vi "GenC37.118Cmd.vi"(7 "Function":T1=enum."Send CFG-2 file", 8 "error in (no error)":errorcluster, 11 "PMUClass":refnum<class "C37.118 PMU.lvclass">) -> (0 "error out":errorcluster, 2 "Command":string, 3 "PMUClass":refnum<class "C37.118 PMU.lvclass">)   [LabVIEW 2018, in "SensorPlugins.lvlib" / "C37.118 PMU.lvclass"]
uses:
  C37.118 PMU.lvclass
  Typedef/eCmdTypes.ctl
  C37.118 PMU.lvclass/C37.118 PMU.ctl
  Accessors/Read PMUComms.vi
panel:
  out "output array":u8[](array[numeric])=[68, 65, 13, 10, 0, 1, 67, 168, 27, 80, 0, 1, 0, 0, 0, 1, 94, 87] format="%x"
  out "*(type *) &x":u8[](array[numeric]) format="%x"
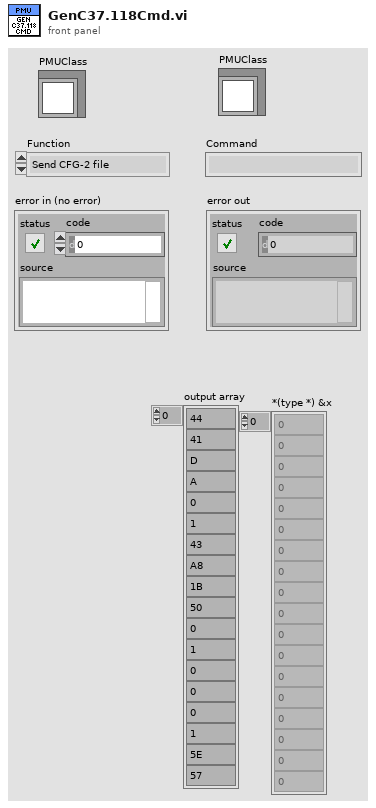
[diagram p1: front panel]
types:
  T1 = typedef "SensorPlugins.lvlib/C37.118 PMU.lvclass/eCmdTypes.ctl" = enum16{"Stop realtime data", "Start realtime data", "Send HDR file", "Send CFG-1 file", "Send CFG-2 file"}
  T2 = typedef "SensorPlugins.lvlib/C37.118 PMU.lvclass/PMUComms.ctl" = cluster{"PMU IP Address":string, "CMD Comms Type":T3, "Data Comms Type":T3, "CMD Port":u16, "Data Port":u16, "PMU ID":u16}
  T3 = typedef "SensorPlugins.lvlib/C37.118 PMU.lvclass/eCommsType.ctl" = enum16{"TCP", "UDP", "USB", "GPIB"}
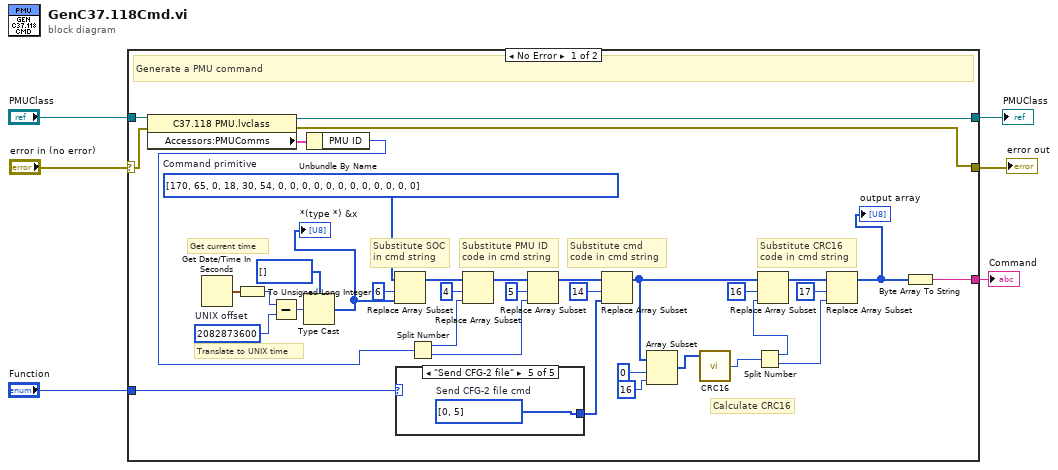
[diagram p0: block diagram]
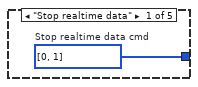
[diagram p2: hidden frame]
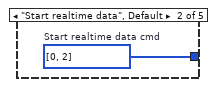
[diagram p3: hidden frame]
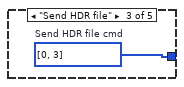
[diagram p4: hidden frame]
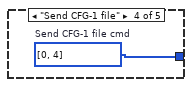
[diagram p5: hidden frame]
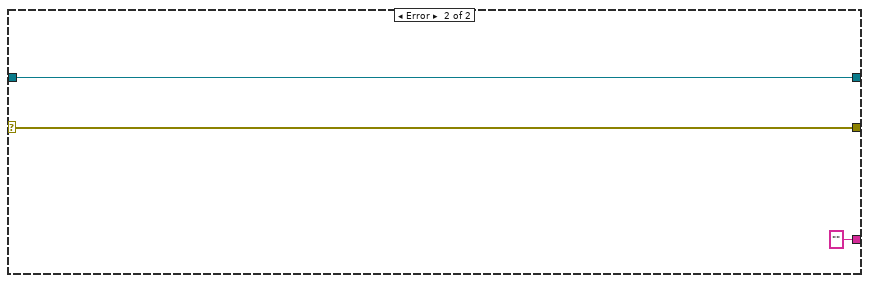
[diagram p6: hidden frame]
diagram:
  n1 = case shown="No Error" "error in (no error)" {
    selector: "error in (no error)" -> [w11 w50]
    tunnel: [w9 w50] -> w5
    tunnel: "PMUClass" -> [w14 w49]
    tunnel: [w10 w49] -> w3
    tunnel: "Function" -> [w8 _]
    tunnel: [w7 "" ("string")] -> w1
    frame No Error {
      w25 = u32 2082873600  # UNIX offset
      w22 = u8[] [170, 65, 0, 18, 30, 54, 0, 0, 0, 0, 0, 0, 0, 0, 0, 0, 0, 0]  # Command primitive
      # "Translate to UNIX time"
      # "Substitute SOC in cmd string"
      # "Get current time"
      # "Calculate CRC16"
      # "Substitute CRC16 code in cmd string"
      # "Substitute cmd code in cmd string"
      # "Substitute PMU ID code in cmd string"
      # "Generate a PMU command"
      n2 = property class="C37.118 PMU.lvclass"(reference=w14, error in=w11) -> (reference out=w10:refnum<class "C37.118 PMU.lvclass">, error out=w9:errorcluster, "Accessors:PMUComms"=w13:T2)
      n3 = Get Date/Time In Seconds() -> (seconds since 1Jan1904=w27:timestamp)
      n4 = To Unsigned Long Integer(number=w27) -> (unsigned 32bit integer=w26:u32)
      n5 = Subtract(x=w26, y=w25) -> (x-y=w24:u32)
      n6 = Type Cast(type=u8[] [], x=w24) -> (*(type *) &x=w18:u8[])
      "*(type *) &x" <- w18
      n7 = Unbundle By Name(w13) -> ("PMU ID"=w12:u16)
      n8 = Replace Array Subset(array=w22, new element=w18, index=6) -> (w21:u8[])
      n9 = case shown="\"Send CFG-2 file\"" w8 {
        tunnel: [w43 w44 w45 w46 w47] -> w15
        frame "Stop realtime data" {
          w43 = u8[] [0, 1]  # Stop realtime data cmd
        }
        frame "Start realtime data", Default {
          w44 = u8[] [0, 2]  # Start realtime data cmd
        }
        frame "Send HDR file" {
          w45 = u8[] [0, 3]  # Send HDR file cmd
        }
        frame "Send CFG-1 file" {
          w46 = u8[] [0, 4]  # Send CFG-1 file cmd
        }
        frame "Send CFG-2 file" {
          w47 = u8[] [0, 5]  # Send CFG-2 file cmd
        }
      }
      n10 = Split Number(x=w12) -> (hi(x)=w32:u8, lo(x)=w28:u8)
      n11 = Replace Array Subset(array=w21, new element=w32, index=4) -> (w30:u8[])
      n12 = Replace Array Subset(array=w30, new element=w28, index=5) -> (w29:u8[])
      n13 = Replace Array Subset(array=w29, new element=w15, index=14) -> (w41:u8[])
      n14 = Array Subset(array=w41, index=0, length=16) -> (w17:u8[])
      n15 = call "CRC16.vi"("Data"=w17) -> ("CRC"=w16:u16)  [unwired: 2 in]
      n16 = Split Number(x=w16) -> (hi(x)=w36:u8, lo(x)=w33:u8)
      n17 = Replace Array Subset(array=w41, new element=w36, index=16) -> (w34:u8[])
      n18 = Replace Array Subset(array=w34, new element=w33, index=17) -> (w19:u8[])
      "output array" <- w19
      n19 = Byte Array To String(unsigned byte array=w19) -> (string=w7:string)
    }
    frame Error {
    }
  }
  "PMUClass" <- w3
  "error out" <- w5
  "Command" <- w1
